vi "stream daemon template.vi"(10 "daemon confg":T1, 11 "module":refnum<class "TBM module execution interface.lvclass">) -> (0 "error out":errorcluster)   [LabVIEW 2013, in "TBM module execution interface.lvclass"]
uses:
  TBM module execution interface.lvclass
  daemon interface.ctl
  <vilib>/NI/Tag Bus/data stream/publisher/publisher.lvclass
  <vilib>/NI/Tag Bus/data stream/subscriber/subscriber.lvclass
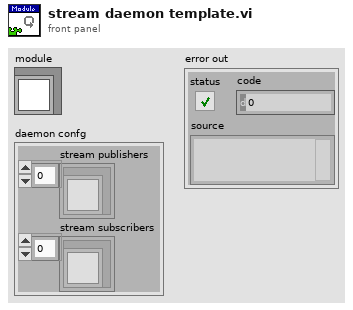
[diagram p1: front panel]
types:
  T1 = typedef "TBM module execution interface.lvclass/daemon interface.ctl" = cluster{"stream publishers":refnum<class "publisher.lvclass">[], "stream subscribers":refnum<class "subscriber.lvclass">[]}
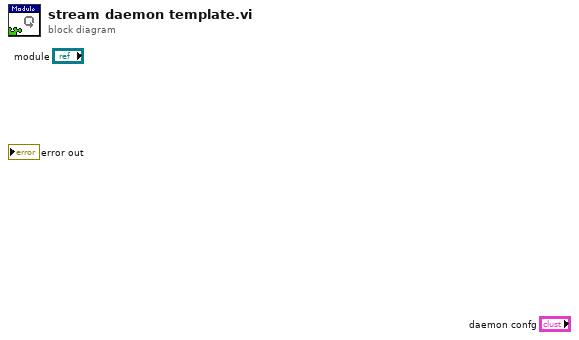
[diagram p0: block diagram]
diagram:
